vi "215.Cleaning cycle (SubVI).vi"(8 "error in (no error)":errorcluster, 9 "Volumen (-1000 to 0)":string="-1000", 10 "milliseconds to wait":u32=7500, 11 "VISA Refnum in":refnum<visa-resource-name>) -> (0 "error out":errorcluster, 1 "Boolean":bool, 3 "VISA out":refnum<visa-resource-name>)   [LabVIEW 2017]
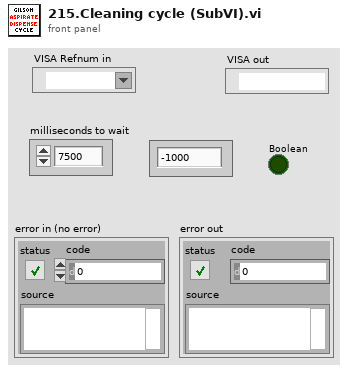
[diagram p1: front panel]
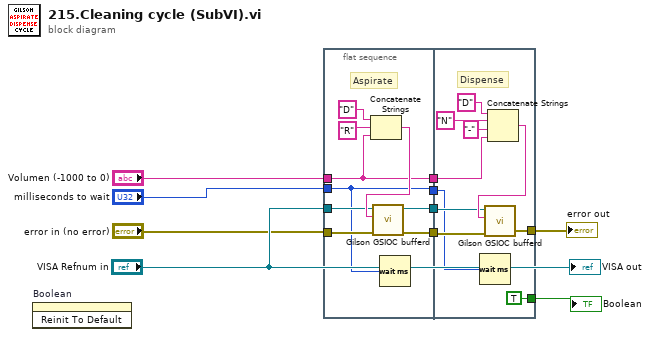
[diagram p0: block diagram]
diagram:
  n1 = invoke on="Boolean" class="Bool (strict)" method="Reinit To Default"() -> ()  [unwired: 3 in, 3 out]
  n2 = flat-sequence {
    tunnel: "VISA Refnum in" -> [w14]
    tunnel: "milliseconds to wait" -> [w12]
    tunnel: [w16] -> w10
    tunnel: [w15] -> w9
    tunnel: [w12] -> w8
    tunnel: "error in (no error)" -> [w13]
    tunnel: [w11] -> w4
    tunnel: "Volumen (-1000 to 0)" -> [w11]
    tunnel: w10 -> [w25]
    tunnel: w9 -> [w26]
    tunnel: w8 -> [w23]
    tunnel: [w24] -> w6
    tunnel: w4 -> [w22]
    tunnel: [TRUE] -> w1
    frame #0 {
      # "Aspirate"
      n3 = Concatenate Strings("D" ("string"), "R" ("string"), w11) -> (w17:string)
      n4 = call <instrlib>:"Gilson GSIOC bufferd.vi"("error in (no error)"=w13, "Bufferd command"=w17, "VISA resource name"=w14) -> ("error out"=w16:errorcluster, "VISA resource name out"=w15:refnum<visa-resource-name>)  [unwired: 6 in, 1 out]
      n5 = Wait (ms)(milliseconds to wait=w12) -> ()  [unwired: 1 out]
    }
    frame #1 {
      # "Dispense"
      n6 = Wait (ms)(milliseconds to wait=w23) -> ()  [unwired: 1 out]
      n7 = Concatenate Strings("D" ("string"), "N" ("string"), "-" ("string"), w22) -> (w27:string)
      n8 = call <instrlib>:"Gilson GSIOC bufferd.vi"("error in (no error)"=w25, "Bufferd command"=w27, "VISA resource name"=w26) -> ("error out"=w24:errorcluster)  [unwired: 6 in, 2 out]
    }
  }
  "error out" <- w6
  "VISA out" <- "VISA Refnum in"
  "Boolean" <- w1
